vi "libssh2_init_default.vi"(8 "error in (no error)":errorcluster, 10 "flags (0 = none)":T1 items=["No Crypto"=1]) -> (0 "error out":errorcluster)   [LabVIEW 2017, in "libssh2.lvlib"]
doc: "Initialize libssh2 with the default build of libssh2 included with lvssh2."
uses:
  libssh2.lvlib
  libssh2_init_flags.ctl
  Global Settings.vi
  libssh2_64.dll
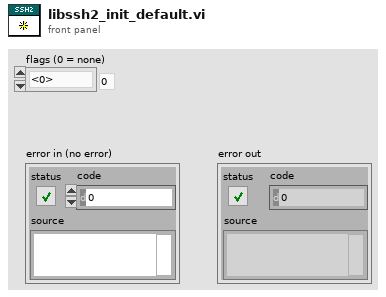
[diagram p1: front panel]
types:
  T1 = typedef "libssh2.lvlib/libssh2_init_flags.ctl" = i32
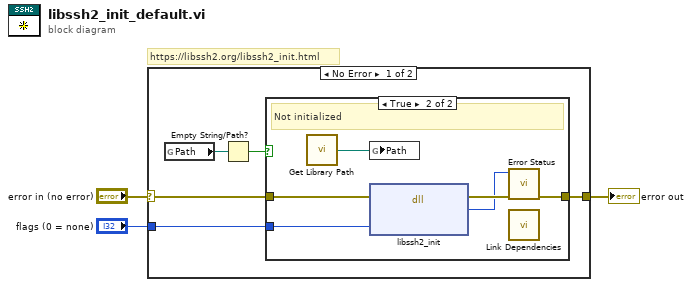
[diagram p0: block diagram]
diagram:
  # "https://libssh2.org/libssh2_init.html"
  n1 = case shown="No Error" "error in (no error)" {
    selector: "error in (no error)" -> [w7 w16]
    tunnel: [w8 w16] -> w3
    tunnel: "flags (0 = none)" -> [w4 _]
    frame No Error {
      n2 = global read "Global Settings.vi" "Path"() -> (w5:path)
      n3 = Empty String/Path?(string/path=w5) -> (empty?=w6:bool)
      n4 = case shown="True" w6 {
        tunnel: [w9 w13] -> w8
        tunnel: w7 -> [w9 w14]
        tunnel: w4 -> [_ w11]
        frame False {
          # "Already initialized"
        }
        frame True {
          # "Not initialized"
          n5 = call "Get Library Path.vi"() -> ("Path"=w10:path)  [unwired: 1 in]
          n6 = global write "Global Settings.vi" "Path"(w10) -> ()
          n7 = dll-call lib="C:/Users/Pascal/Projects/Home/lvssh2/libssh2/libssh2**.*" fn="libssh2_init"(error in=w14, "flags"=w11) -> (error out=w15:errorcluster, "return value"=w12:i32)  [unwired: 3 in, 1 out]
          n8 = call "Error Status.vi"("error in (no error)"=w15, "return value"=w12) -> ("error out"=w13:errorcluster)  [unwired: 8 in, 1 out]
          n9 = call "Link Dependencies.vi"() -> ()  [unwired: 12 in]
        }
      }
    }
    frame Error {
    }
  }
  "error out" <- w3
